vi "Configure Protect Volt.vi"(7 "Volt Delay(0)":dbl min=0.0 max=300.0, 8 "error in (no error)":errorcluster, 9 "Volt(0)":dbl min=0.0 max=300.0, 10 "Enable":bool, 11 "VISA resource name":refnum<visa-resource-name>) -> (0 "error out":errorcluster, 3 "VISA resource name out":refnum<visa-resource-name>)   [LabVIEW 2020, in "IT6500.lvlib"]
doc: "This command is used to set the software voltage protection value of the power supply."
uses:
  IT6500.lvlib
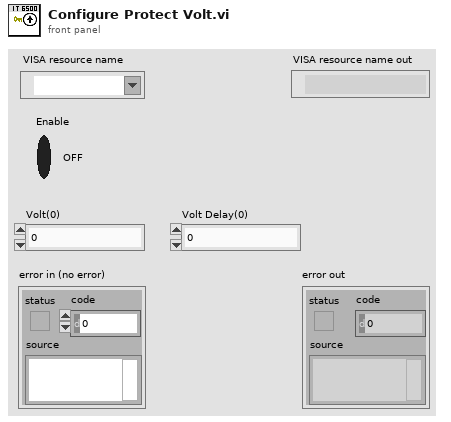
[diagram p1: front panel]
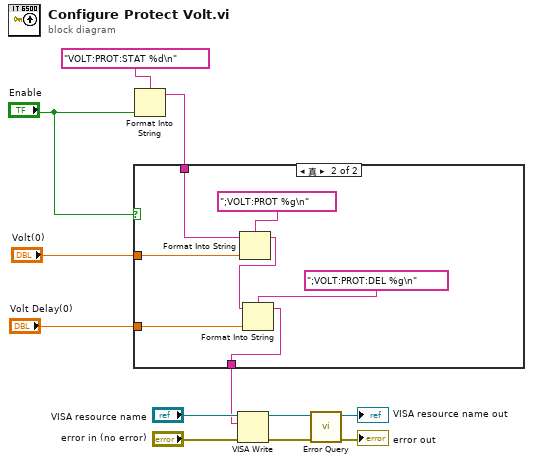
[diagram p0: block diagram]
diagram:
  n1 = Format Into String(format string="VOLT:PROT:STAT %d\n", "Enable") -> (resulting string=w5:string)  [unwired: 2 in, 1 out]
  n2 = case shown="真" "Enable" {
    tunnel: w5 -> [w13 w18]
    tunnel: "Volt(0)" -> [_ w20]
    tunnel: [w13 w16] -> w2
    tunnel: "Volt Delay(0)" -> [_ w15]
    frame False {
    }
    frame True {
      n3 = Format Into String(format string=";VOLT:PROT %g\n", initial string=w18, w20) -> (resulting string=w17:string)  [unwired: 1 in, 1 out]
      n4 = Format Into String(format string=";VOLT:PROT:DEL %g\n", initial string=w17, w15) -> (resulting string=w16:string)  [unwired: 1 in, 1 out]
    }
  }
  n5 = VISA Write(VISA resource name="VISA resource name", write buffer=w2, error in (no error)="error in (no error)") -> (VISA resource name out=w9:refnum<visa-resource-name>, error out=w10:errorcluster)  [unwired: 1 out]
  n6 = call "Error Query.vi"("error in (no error)"=w10, "VISA resource name"=w9) -> ("error out"=→"error out":errorcluster, "VISA resource name out"=→"VISA resource name out":refnum<visa-resource-name>)  [unwired: 6 in, 2 out]
